vi "UTILITY Agilent Scan List Permutation.vi"(8 "Error In":errorcluster, 9 "Input Data Array":dbl[](array[numeric]), 10 "Agilent Scan List":string="111,112,113,114,115,116,109,110,313,201,202,203,204,205,206,207,208,209,210,211,212,213,214,215,216,107,108,314,315,316,105,106,301,302,303,304,305,306,307,308,309,310,311,312,101,102,103,104") -> (0 "Error Out":errorcluster, 1 "Output Data Permutation":dbl[](array[numeric]), 2 "Names":string[](array[string]))   [LabVIEW 2018]
panel:
  out "size(s)":i32
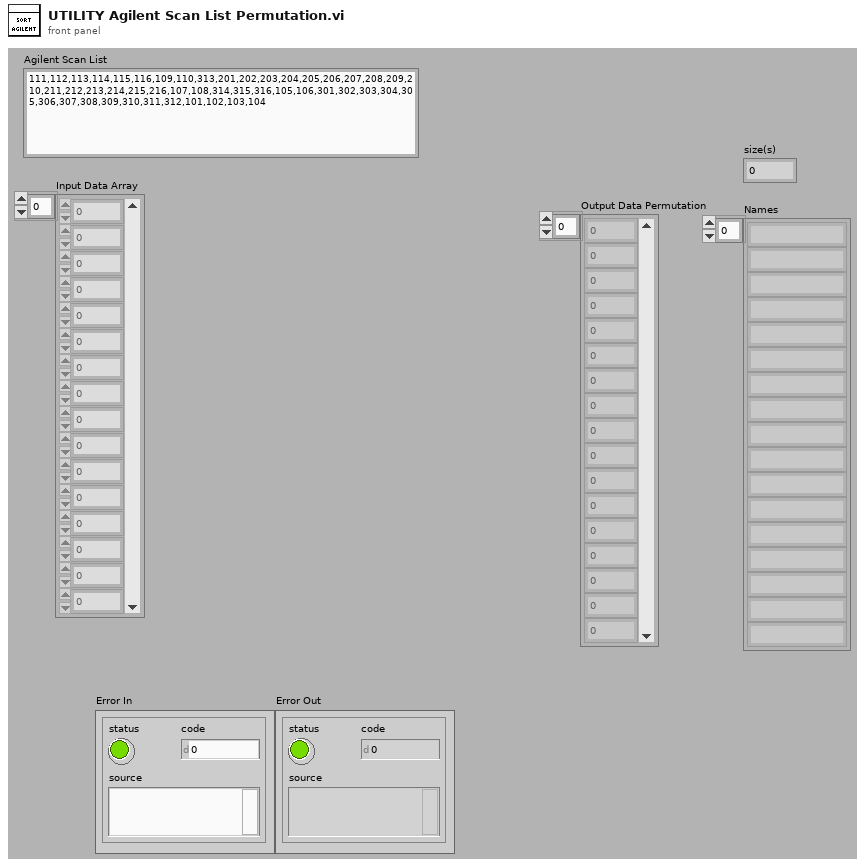
[diagram p1: front panel]
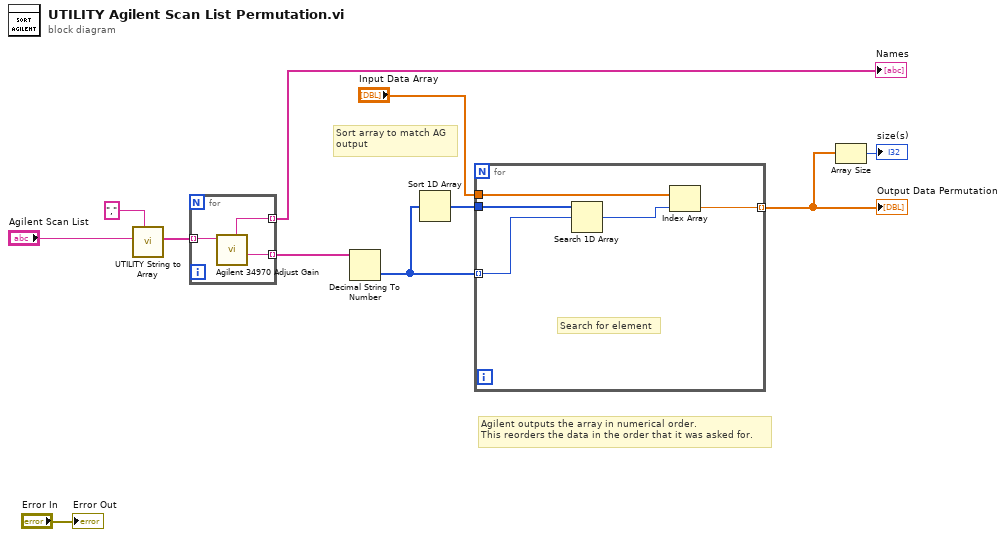
[diagram p0: block diagram]
diagram:
  # "Sort array to match AG\noutput"
  # "Agilent outputs the array in numerical order. \nThis reorders the data in the order that it was asked for."
  n1 = call "UTILITY String to Array.vi"("Delimiter"=",", "String"="Agilent Scan List") -> ("Array"=w4:string[])  [unwired: 9 in]
  n2 = for {
    tunnel: w4 -> [w14] mode=indexing
    tunnel: [w13] -> w3 mode=indexing
    tunnel: [w12] -> w2 mode=indexing
    n3 = call "Agilent 34970 Adjust Gain.vi"("Input Channel"=w14) -> ("Output Channel"=w13:string, "Name"=w12:string)  [unwired: 6 in, 3 out]
  }
  "Names" <- w2
  n4 = Decimal String To Number(string=w3) -> (number=w1:i32[])  [unwired: 2 in, 1 out]
  n5 = Sort 1D Array(array=w1) -> (sorted array=w8:i32[])
  n6 = for {
    tunnel: "Input Data Array" -> [w19]
    tunnel: [w18] -> w6 mode=indexing
    tunnel: w8 -> [w16]
    tunnel: w1 -> [w15] mode=indexing
    # "Search for element"
    n7 = Search 1D Array(1D array=w16, element=w15) -> (index of element=w17:i32)  [unwired: 1 in]
    n8 = Index Array(array=w19, index=w17) -> (element=w18:dbl)
  }
  "Output Data Permutation" <- w6
  n9 = Array Size(array=w6) -> (size(s)=→"size(s)":i32)
  "Error Out" <- "Error In"
